vi "LED-Testing-JAP_v8.vi"() -> ()   [LabVIEW 2018]
uses:
  <vilib>/Utility/file.llb/Write Delimited Spreadsheet (string).vi
  LED_Test_JAP/SubVIs_LED-Testing-JAP_v2/Keithley 24XX/Keithley 24XX.lvlib
panel:
  in  "Compl. 3 (A)":dbl=0.09
  in  "Volt for Comp. 3 (V)":dbl=4.0 format="%#_13g"
  in  "Compl. 1 (A)":dbl=0.0009
  in  "Compl. 2 (A)":dbl=0.009
  out "Test Current (A)":string
  in  "Test":bool
  in  "stop":bool
  in  "Test Voltage (V)":dbl=0.1
  in  "Voltage range (V)":enum16{"0.2", "2", "20", "200"}(ring)=enum."20"
  out "Spectrum":cluster{"Y":dbl[], "Y":dbl[]}[](graph)
  out "L-V":cluster{"Y":dbl[], "Y":dbl[]}[](graph)
  out "Current efficiency - V":cluster{"Y":dbl[], "Y":dbl[]}[](graph)
  in  "Step 2 (V)":dbl=0.5 format="%#_13g"
  in  "End (V)":dbl=15.0 format="%#_13g"
  out "Voltage (V) 2":dbl
  out "Current (A) 2":string
  out "Exp. Meas. Time 2":string
  out "Meas. complete 2":string
  out "Data - x, y, Lv 2":dbl[](array[numeric])
  out "Spectrum (380-780nm) 2":dbl[](array[numeric])
  in  "Mode 2":enum16{"iV", "iVL"}(ring)=enum."iVL"
  in  "Interval 2 (ms)":dbl=500.0
  in  "Mode 1":enum16{"iV", "iVL"}(ring)
  in  "?":enum32{"Results", "Spectra"}(tab)
  out "Area (mm2), Voltage (V),  Current (A), Current density (mA/cm2), Current efficiency (Cd/A), Luminance (Cd/m2), CIEx, CIEy":ext[][](array[numeric])
  out "Spectral radiant intensity at different voltages (header)":ext[][](array[numeric])
  out "Spectrum (380-780nm)":dbl[](array[numeric])
  out "Data - x, y, Lv":dbl[](array[numeric])
  out "Meas. complete":string
  out "Exp. Meas. Time":string
  in  "error in (no error)":errorcluster
  in  "CS-2000 VISA name":refnum<visa-resource-name>="COM3"
  out "error out 2":errorcluster
  in  "Compliance (A)":dbl=0.0009
  in  "Start (V)":dbl
  in  "Mid (V)":dbl=2.5 format="%#_13g"
  in  "Step 1 (V)":dbl=0.1 format="%#_13g"
  out "Voltage (V)":dbl
  out "Current (A)":string
  in  "Stop":bool
  out "J-V":cluster{"Y":dbl[], "Y":dbl[]}[](graph)
  in  "Pixel area (mm2)":dbl=4.5
  in  "Interval 1 (ms)":dbl=500.0
  in  "Directory:":path=path "C:/Users/Talapin Lab/Desktop/LED_Test_JAP/Data/Himchan/20180725"
  in  "File name:":string
  in  "Insert time stamp:":bool=TRUE
  in  "Quit":bool
  in  "Start":bool
  in  "Keithley2400 VISA name":refnum<visa-resource-name>="GPIB0::24::INSTR"
  # "Area (mm2)"
  # "Voltage (V)"
  # "Current (A)"
  # "Current density (mA/cm2)"
  # "Current efficiency (Cd/A)"
  # "Luminance \n(Cd/m2)"
  # "CIEx"
  # "CIEy"
  # "Wavelength (nm)"
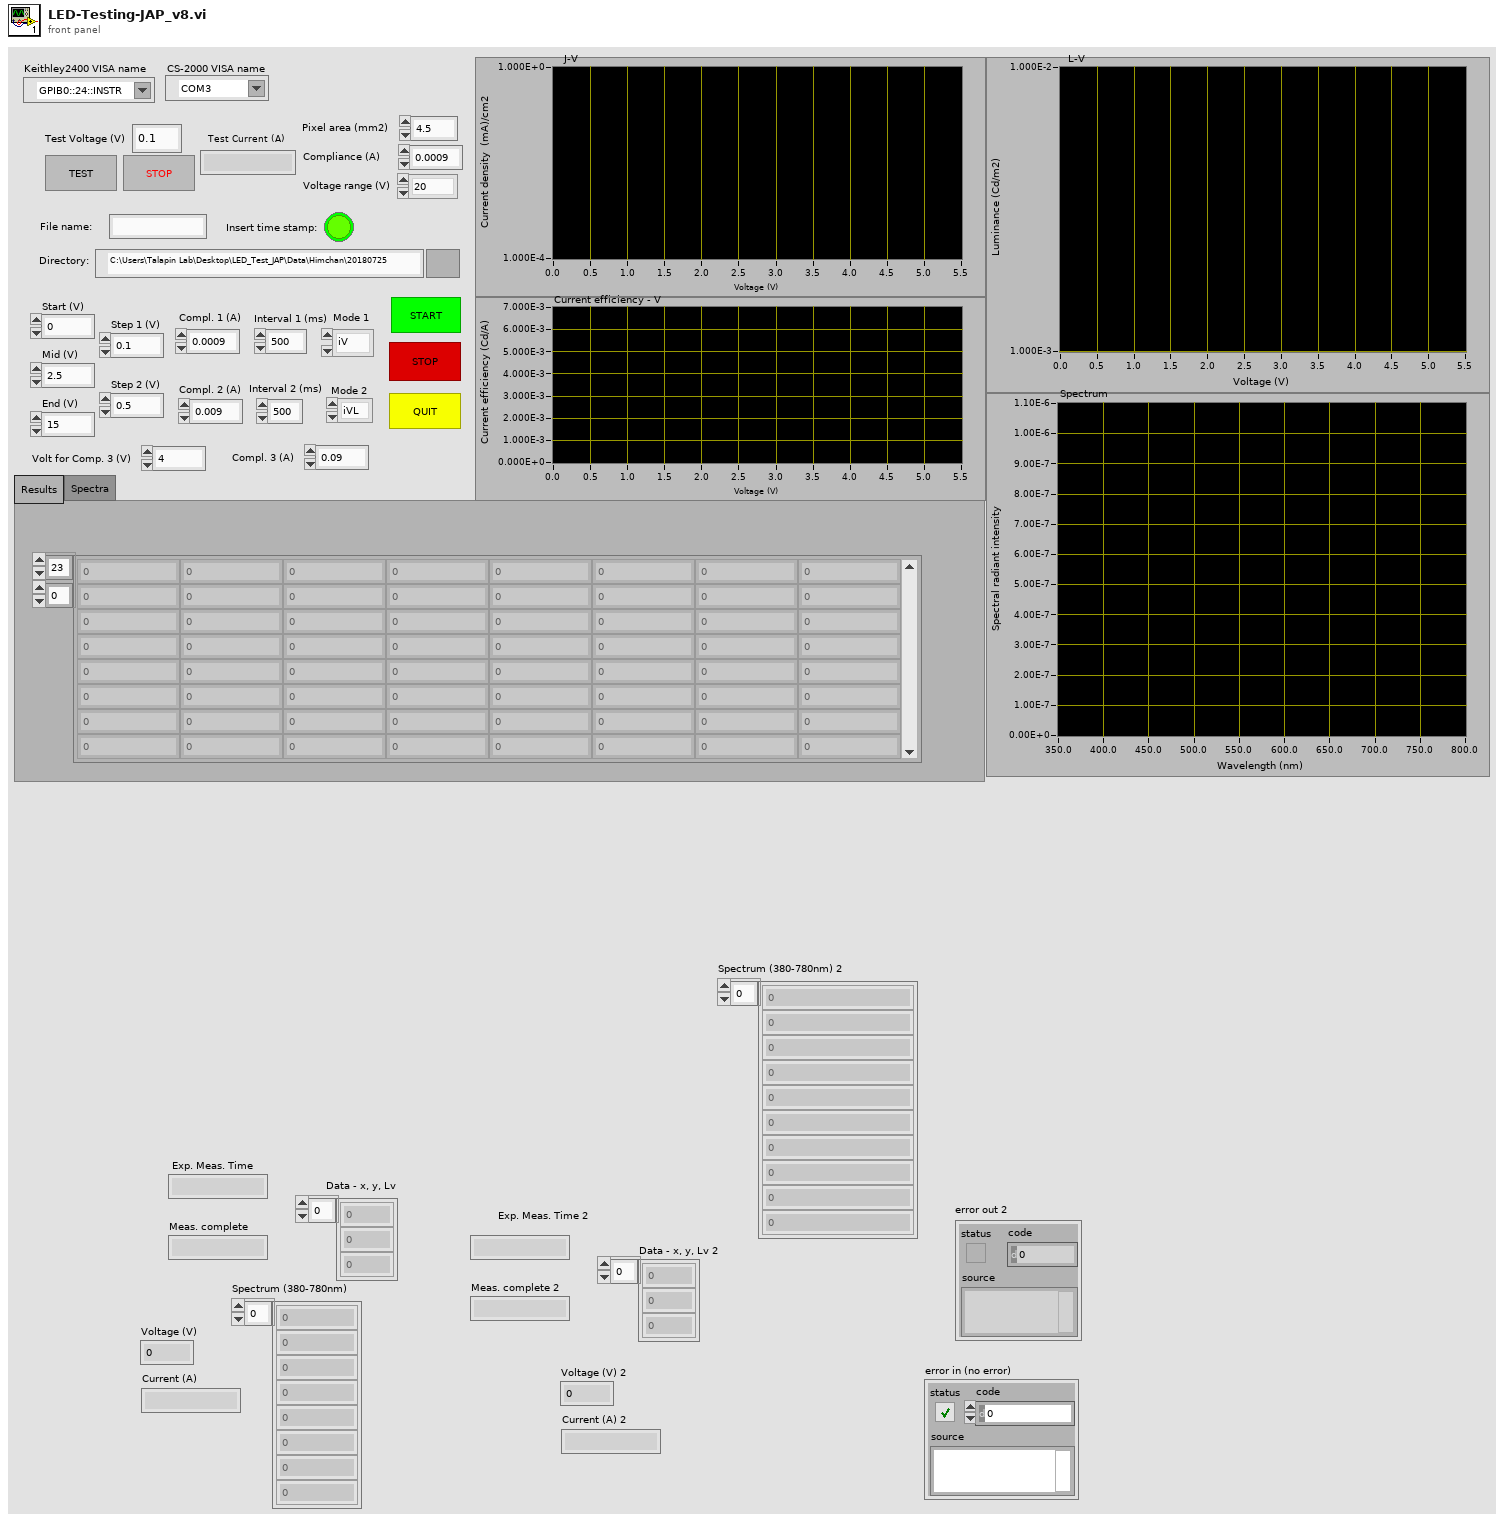
[diagram p1: front panel]
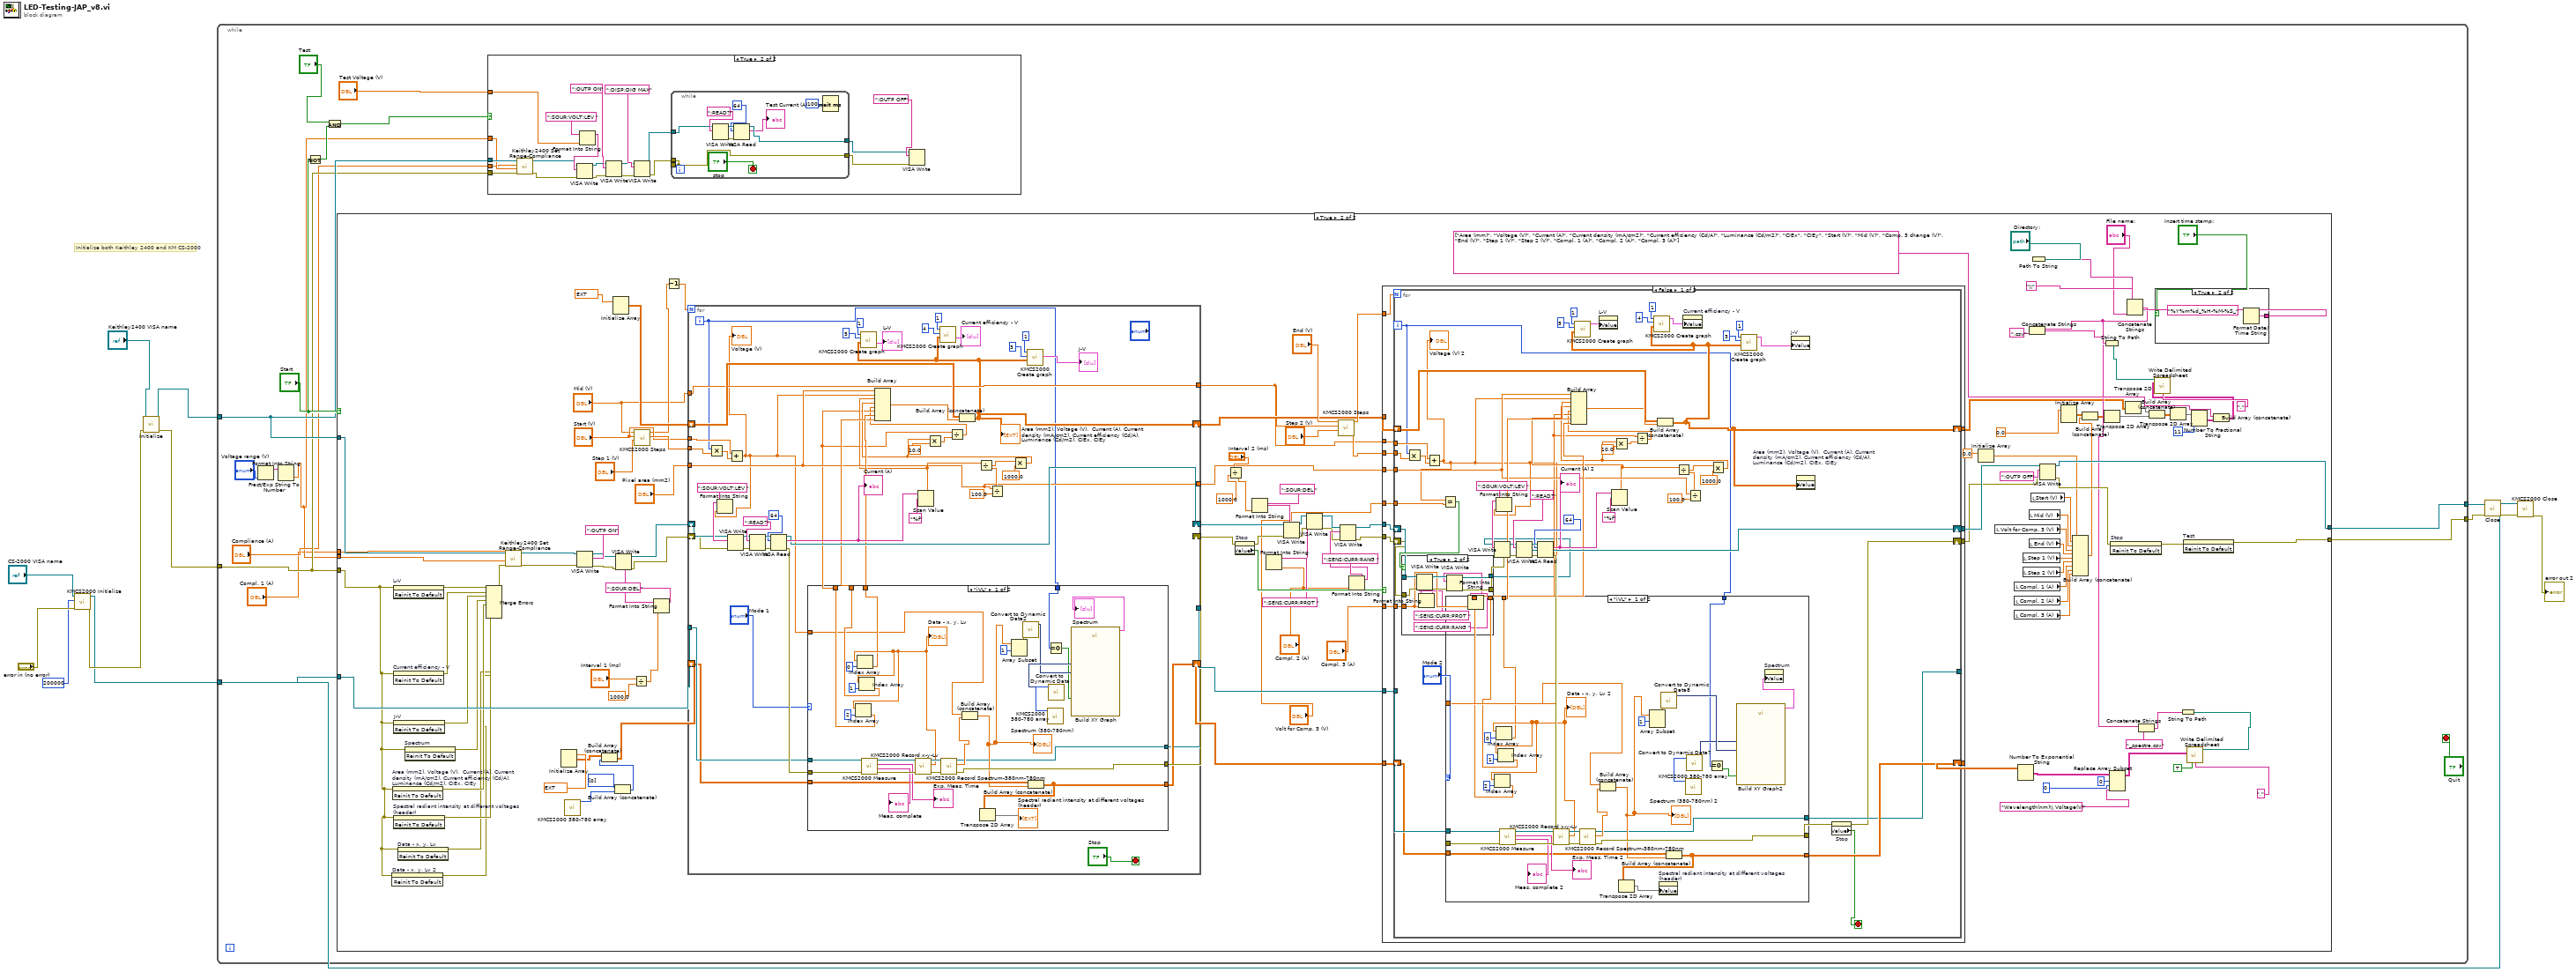
[diagram p0: block diagram]
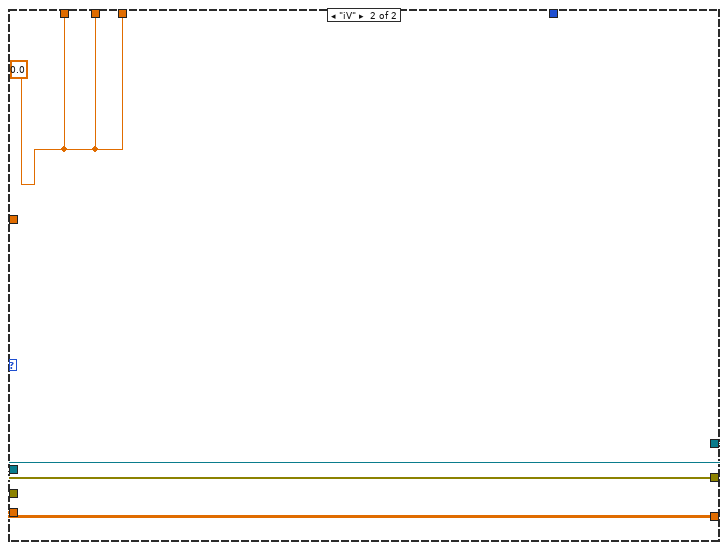
[diagram p5: hidden frame]
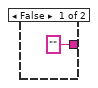
[diagram p7: hidden frame]
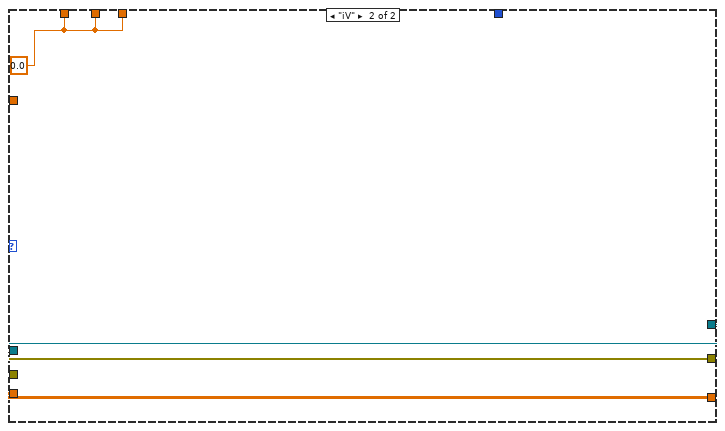
[diagram p8: hidden frame]
diagram:
  # "Initialize both Keithley 2400 and KM CS-2000"
  n1 = call "KMCS2000 Initialize.vi"("error in (no error)"="error in (no error)", "timeout (10sec)"=u32 200000, "VISA Refnum in"="CS-2000 VISA name") -> ("error out"=w5:errorcluster, "VISA Refnum out"=w2:refnum<visa-resource-name>)  [unwired: 7 in]
  n2 = call "Initialize.vi"("error in (no error)"=w5, "VISA resource name"="Keithley2400 VISA name") -> ("error out"=w10:errorcluster, "VISA resource name out"=w11:refnum<visa-resource-name>)  [unwired: 8 in]
  n3 = while {
    tunnel: w11 -> [w21]
    tunnel: w10 -> [w20]
    tunnel: [w28] -> w9
    tunnel: [w27] -> w8
    tunnel: w2 -> [w25]
    stop <- "Quit" stop-if-true
    n4 = Format Into String("Voltage range (V)") -> (resulting string=w17:string)  [unwired: 3 in, 1 out]
    n5 = Fract/Exp String To Number(string=w17) -> (number=w16:dbl)  [unwired: 3 in, 1 out]
    n6 = Not(x="Start") -> (.not. x?=w23:bool)
    n7 = And(x="Test", y=w23) -> (x .and. y?=w22:bool)
    n8 = case shown="True" "Start" {
      tunnel: w21 -> [w60 w185]
      tunnel: w20 -> [w59 w87]
      tunnel: [w60 w178] -> w28
      tunnel: [w59 w106] -> w27
      tunnel: w25 -> [_ w155]
      tunnel: w16 -> [_ w109]
      tunnel: "Compl. 1 (A)" -> [_ w108]
      frame False {
      }
      frame True {
        n9 = invoke on="Data - x, y, Lv 2" class="Arr (strict)" method="Reinit To Default"(error in=w87) -> (error out=w85:errorcluster)  [unwired: 2 in, 2 out]
        n10 = invoke on="Area (mm2), Voltage (V),  Current (A), Current density (mA/cm2), Current efficiency (Cd/A), Luminance (Cd/m2), CIEx, CIEy" class="Arr (strict)" method="Reinit To Default"(error in=w87) -> (error out=w100:errorcluster)  [unwired: 2 in, 2 out]
        n11 = invoke on="L-V" class="XYGraph (strict)" method="Reinit To Default"(error in=w87) -> (error out=w104:errorcluster)  [unwired: 2 in, 2 out]
        n12 = invoke on="Current efficiency - V" class="XYGraph (strict)" method="Reinit To Default"(error in=w87) -> (error out=w103:errorcluster)  [unwired: 2 in, 2 out]
        n13 = invoke on="J-V" class="XYGraph (strict)" method="Reinit To Default"(error in=w87) -> (error out=w102:errorcluster)  [unwired: 2 in, 2 out]
        n14 = invoke on="Spectral radiant intensity at different voltages (header)" class="Arr (strict)" method="Reinit To Default"(error in=w87) -> (error out=w99:errorcluster)  [unwired: 2 in, 2 out]
        n15 = invoke on="Data - x, y, Lv" class="Arr (strict)" method="Reinit To Default"(error in=w87) -> (error out=w86:errorcluster)  [unwired: 2 in, 2 out]
        n16 = invoke on="Spectrum" class="XYGraph (strict)" method="Reinit To Default"(error in=w87) -> (error out=w101:errorcluster)  [unwired: 2 in, 2 out]
        n17 = Merge Errors(w104, w103, w102, w101, w100, w99, w86, w85) -> (w105:errorcluster)
        n18 = call "Keithley2400 Set Range-Compliance.vi"("error in (no error)"=w105, "Voltage range (V)"=w109, "Compliance (A)"=w108, "VISA Refnum in"=w185) -> ("error out"=w166:errorcluster, "VISA Refnum out"=w171:refnum<visa-resource-name>)  [unwired: 6 in]
        n19 = Initialize Array(ext 0.0) -> (w153:ext[][])  [unwired: 2 out]
        n20 = call "KMCS2000 380-780 array.vi"() -> ("Array"=w144:i32[])  [unwired: 11 in]
        n21 = VISA Write(VISA resource name=w171, write buffer=":OUTP ON", error in (no error)=w166) -> (VISA resource name out=w170:refnum<visa-resource-name>, error out=w167:errorcluster)  [unwired: 1 out]
        n22 = Initialize Array(ext 0.0) -> (w180:ext[][])  [unwired: 2 out]
        n23 = Build Array (concatenate)(i32[] [0] ("array"), w144) -> (w145:i32[])
        n24 = Build Array (concatenate)(w153, w145) -> (w152:ext[][])
        n25 = Divide(x="Interval 1 (ms)", y=1000.0) -> (x/y=w174:dbl)
        n26 = call "KMCS2000 Steps.vi"("Step 1"="Step 1 (V)", "Start (V)"="Start (V)", "Mid (V)"="Mid (V)") -> ("Step sizeand direction"=w183:dbl, "Number of steps"=w117:dbl)  [unwired: 7 in]
        n27 = Format Into String(initial string=":SOUR:DEL " ("write buffer"), w174) -> (resulting string=w175:string)  [unwired: 2 in, 1 out]
        n28 = VISA Write(VISA resource name=w170, write buffer=w175, error in (no error)=w167) -> (VISA resource name out=w169:refnum<visa-resource-name>, error out=w168:errorcluster)  [unwired: 1 out]
        n29 = Decrement(x=w117) -> (x-1=w116:dbl)
        n30 = for {
          N: w116 -> [_]
          tunnel: w183 -> [w364]
          tunnel: "Start (V)" -> [w333]
          shift-right: [w315] -> w122
          shift-left: w180 -> [w362]
          shift-right: [w351] -> w130
          shift-left: w169 -> [w353]
          shift-right: [w340] -> w112
          shift-left: w168 -> [w352]
          tunnel: w155 -> [w341]
          shift-right: [w336] -> w124
          shift-left: w152 -> [w337]
          tunnel: "Pixel area (mm2)" -> [w330]
          tunnel: [w335] -> w123
          tunnel: [w330] -> w129
          tunnel: [w332] -> w118
          tunnel: "Mid (V)" -> [w332]
          i -> [w313]
          stop <- "Stop" stop-if-true
          n31 = Multiply(x=w313, y=w364) -> (x*y=w363:dbl)
          n32 = Add(x=w333, y=w363) -> (x+y=w329:dbl)
          "Voltage (V)" <- w329
          n33 = Format Into String(initial string=":SOUR:VOLT:LEV " ("write buffer"), w329) -> (resulting string=w359:string)  [unwired: 2 in, 1 out]
          n34 = VISA Write(VISA resource name=w353, write buffer=w359, error in (no error)=w352) -> (VISA resource name out=w354:refnum<visa-resource-name>, error out=w350:errorcluster)  [unwired: 1 out]
          n35 = VISA Write(VISA resource name=w354, write buffer=":READ?", error in (no error)=w350) -> (VISA resource name out=w357:refnum<visa-resource-name>, error out=w349:errorcluster)  [unwired: 1 out]
          n36 = VISA Read(VISA resource name=w357, byte count=u32 64, error in (no error)=w349) -> (VISA resource name out=w351:refnum<visa-resource-name>, read buffer=w356:string, error out=w342:errorcluster)  [unwired: 1 out]
          "Current (A)" <- w356
          n37 = case shown="\"iVL\"" "Mode 1" {
            tunnel: w342 -> [w386 w398]
            tunnel: w341 -> [w385 w396]
            tunnel: [w384 w398] -> w340
            tunnel: [w379 w399] -> w325
            tunnel: [w378 w399] -> w339
            tunnel: [w377 w399] -> w338
            tunnel: w337 -> [w376 w397]
            tunnel: [w375 w397] -> w336
            tunnel: w329 -> [w372 _]
            tunnel: [w368 w396] -> w335
            tunnel: w313 -> [w365 _]
            frame "iVL" {
              n38 = call "KMCS2000 Measure.vi"("error in (no error)"=w386, "VISA Refnum in"=w385) -> ("error out"=w394:errorcluster, "Meas. complete"=→"Meas. complete":string, "Exp. Meas. Time"=→"Exp. Meas. Time":string, "VISA Refnum out"=w395:refnum<visa-resource-name>)  [unwired: 6 in]
              n39 = call "KMCS2000 Record x-y-Lv.vi"("error in (no error)"=w394, "VISA Refnum in"=w395) -> ("error out"=w392:errorcluster, "Data - x, y, Lv"=w380:dbl[], "VISA Refnum out"=w393:refnum<visa-resource-name>)  [unwired: 7 in]
              "Data - x, y, Lv" <- w380
              n40 = Index Array(array=w380, index=2) -> (element=w379:dbl)
              n41 = Index Array(array=w380, index=0) -> (element=w378:dbl)
              n42 = Index Array(array=w380, index=1) -> (element=w377:dbl)
              n43 = call "KMCS2000 Record Spectrum-380nm-780nm.vi"("error in (no error)"=w392, "VISA Refnum in"=w393) -> ("error out"=w384:errorcluster, "Spectrum (380-780nm)"=w373:dbl[], "VISA Refnum out"=w368:refnum<visa-resource-name>)  [unwired: 7 in]
              n44 = Build Array (concatenate)(w372, w373) -> (w371:dbl[])
              "Spectrum (380-780nm)" <- w371
              n45 = Array Subset(array=w371, index=1) -> (w370:dbl[])  [unwired: 1 in]
              n46 = call "Convert to Dynamic Data2"("Array"=w370) -> ("Dynamic Data Type"=w387:dynamicdata)  [unwired: 3 in]
              n47 = Build Array (concatenate)(w376, w371) -> (w375:ext[][])
              n48 = Transpose 2D Array(2D array=w375) -> (transposed array=→"Spectral radiant intensity at different voltages (header)":ext[][])
              n49 = call "KMCS2000 380-780 array.vi"() -> ("Array"=w389:i32[])  [unwired: 11 in]
              n50 = Equal To 0?(x=w365) -> (x = 0?=w366:bool)
              n51 = call "Convert to Dynamic Data"("Array"=w389) -> ("Dynamic Data Type"=w388:dynamicdata)  [unwired: 3 in]
              n52 = call "Build XY Graph"("Reset"=w366, "Y Input"=w387, "X Input"=w388) -> ("XY Graph"=→"Spectrum":cluster{"X":dbl[], "Y":dbl[]}[])  [unwired: 7 in, 1 out]
            }
            frame "iV" {
              w399 = 0.0
            }
          }
          n53 = Scan Value(string=w356, format string="%f") -> (value=w328:dbl)  [unwired: 1 in, 1 out]
          n54 = Divide(x=w330, y=100.0) -> (x/y=w345:dbl)
          n55 = Divide(x=w328, y=w345) -> (x/y=w344:dbl)
          n56 = Multiply(x=w344, y=1000.0) -> (x*y=w327:dbl)
          n57 = Multiply(x=w327, y=10.0) -> (x*y=w324:dbl)
          n58 = Divide(x=w325, y=w324) -> (x/y=w323:dbl)
          n59 = Build Array(w330, w329, w328, w327, w323, w325, w339, w338) -> (w361:dbl[])
          n60 = Build Array (concatenate)(w362, w361) -> (w315:ext[][])
          "Area (mm2), Voltage (V),  Current (A), Current density (mA/cm2), Current efficiency (Cd/A), Luminance (Cd/m2), CIEx, CIEy" <- w315
          n61 = call "KMCS2000 Create graph.vi"("Array"=w315, "y index"=5 ("disabled index (col)"), "x index"=1 ("disabled index (col)")) -> ("XY Graph"=→"L-V":cluster{"X":dbl[], "Y":dbl[]}[])  [unwired: 8 in]
          n62 = call "KMCS2000 Create graph.vi"("Array"=w315, "y index"=4 ("disabled index (col)"), "x index"=1 ("disabled index (col)")) -> ("XY Graph"=→"Current efficiency - V":cluster{"X":dbl[], "Y":dbl[]}[])  [unwired: 8 in]
          n63 = call "KMCS2000 Create graph.vi"("Array"=w315, "y index"=3 ("disabled index (col)"), "x index"=1 ("disabled index (col)")) -> ("XY Graph"=→"J-V":cluster{"X":dbl[], "Y":dbl[]}[])  [unwired: 8 in]
        }
        n64 = Divide(x="Interval 2 (ms)", y=1000.0) -> (x/y=w134:dbl)
        n65 = property on="Stop" class="Bool (strict)"(error in=w112) -> (error out=w111:errorcluster, "Value"=w110:bool)  [unwired: 1 in, 1 out]
        n66 = Format Into String(initial string=":SOUR:DEL " ("write buffer"), w134) -> (resulting string=w131:string)  [unwired: 2 in, 1 out]
        n67 = Format Into String(initial string=":SENS:CURR:PROT " ("write buffer"), "Compl. 2 (A)") -> (resulting string=w96:string)  [unwired: 2 in, 1 out]
        n68 = VISA Write(VISA resource name=w130, write buffer=w131, error in (no error)=w111) -> (VISA resource name out=w91:refnum<visa-resource-name>, error out=w89:errorcluster)  [unwired: 1 out]
        n69 = VISA Write(VISA resource name=w91, write buffer=w96, error in (no error)=w89) -> (VISA resource name out=w93:refnum<visa-resource-name>, error out=w92:errorcluster)  [unwired: 1 out]
        n70 = call "KMCS2000 Steps.vi"("Step 1"="Step 2 (V)", "Start (V)"=w118, "Mid (V)"="End (V)") -> ("Step sizeand direction"=w126:dbl, "Number of steps"=w125:dbl)  [unwired: 7 in]
        n71 = Format Into String(initial string=":SENS:CURR:RANG " ("write buffer"), "Compl. 2 (A)") -> (resulting string=w95:string)  [unwired: 2 in, 1 out]
        n72 = VISA Write(VISA resource name=w93, write buffer=w95, error in (no error)=w92) -> (VISA resource name out=w90:refnum<visa-resource-name>, error out=w88:errorcluster)  [unwired: 1 out]
        n73 = case shown="False" w110 {
          tunnel: w129 -> [w200 _]
          tunnel: w126 -> [w199 _]
          tunnel: w125 -> [w198 _]
          tunnel: w124 -> [w197 w308]
          tunnel: w123 -> [w196 _]
          tunnel: w122 -> [w195 w309]
          tunnel: [w194 w309] -> w65
          tunnel: [w193 w306] -> w121
          tunnel: [w192 w307] -> w120
          tunnel: [w191 w308] -> w119
          tunnel: w118 -> [w190 _]
          tunnel: w90 -> [w189 w306]
          tunnel: w88 -> [w188 w307]
          tunnel: "Volt for Comp. 3 (V)" -> [w187 _]
          tunnel: "Compl. 3 (A)" -> [w186 _]
          frame False {
            n74 = for {
              N: w198 -> [_]
              tunnel: w199 -> [w257]
              tunnel: w190 -> [w256]
              shift-right: [w213] -> w194
              shift-left: w195 -> [w254]
              shift-right: [w244] -> w193
              shift-left: w189 -> [w205]
              shift-right: [w222] -> w192
              shift-left: w188 -> [w203]
              tunnel: w196 -> [w236]
              shift-right: [w232] -> w191
              shift-left: w197 -> [w233]
              tunnel: w200 -> [w229]
              tunnel: [w231] -> _
              tunnel: w187 -> [w207]
              tunnel: w186 -> [w201]
              i -> [w209]
              stop <- w220 stop-if-true
              n75 = Multiply(x=w209, y=w257) -> (x*y=w255:dbl)
              n76 = Add(x=w256, y=w255) -> (x+y=w208:dbl)
              "Voltage (V) 2" <- w208
              n77 = Equal?(x=w208, y=w207) -> (x = y?=w206:bool)
              n78 = case shown="True" w206 {
                tunnel: w205 -> [w259 w270]
                tunnel: [w259 w268] -> w204
                tunnel: w203 -> [w258 w267]
                tunnel: [w258 w265] -> w202
                tunnel: w201 -> [_ w264]
                frame False {
                }
                frame True {
                  n79 = Format Into String(initial string=":SENS:CURR:PROT " ("write buffer"), w264) -> (resulting string=w262:string)  [unwired: 2 in, 1 out]
                  n80 = VISA Write(VISA resource name=w270, write buffer=w262, error in (no error)=w267) -> (VISA resource name out=w269:refnum<visa-resource-name>, error out=w266:errorcluster)  [unwired: 1 out]
                  n81 = Format Into String(initial string=":SENS:CURR:RANG " ("write buffer"), w264) -> (resulting string=w260:string)  [unwired: 2 in, 1 out]
                  n82 = VISA Write(VISA resource name=w269, write buffer=w260, error in (no error)=w266) -> (VISA resource name out=w268:refnum<visa-resource-name>, error out=w265:errorcluster)  [unwired: 1 out]
                }
              }
              n83 = Format Into String(initial string=":SOUR:VOLT:LEV " ("write buffer"), w208) -> (resulting string=w251:string)  [unwired: 2 in, 1 out]
              n84 = VISA Write(VISA resource name=w204, write buffer=w251, error in (no error)=w202) -> (VISA resource name out=w245:refnum<visa-resource-name>, error out=w243:errorcluster)  [unwired: 1 out]
              n85 = VISA Write(VISA resource name=w245, write buffer=":READ?", error in (no error)=w243) -> (VISA resource name out=w249:refnum<visa-resource-name>, error out=w242:errorcluster)  [unwired: 1 out]
              n86 = VISA Read(VISA resource name=w249, byte count=u32 64, error in (no error)=w242) -> (VISA resource name out=w244:refnum<visa-resource-name>, read buffer=w247:string, error out=w237:errorcluster)  [unwired: 1 out]
              "Current (A) 2" <- w247
              n87 = case shown="\"iVL\"" "Mode 2" {
                tunnel: w237 -> [w294 w304]
                tunnel: w236 -> [w293 w302]
                tunnel: [w292 w304] -> w221
                tunnel: [w287 w305] -> w224
                tunnel: [w286 w305] -> w235
                tunnel: [w285 w305] -> w234
                tunnel: w233 -> [w284 w303]
                tunnel: [w283 w303] -> w232
                tunnel: w208 -> [w281 _]
                tunnel: [w277 w302] -> w231
                tunnel: w209 -> [w272 _]
                frame "iVL" {
                  n88 = call "KMCS2000 Measure.vi"("error in (no error)"=w294, "VISA Refnum in"=w293) -> ("error out"=w300:errorcluster, "Meas. complete"=→"Meas. complete 2":string, "Exp. Meas. Time"=→"Exp. Meas. Time 2":string, "VISA Refnum out"=w301:refnum<visa-resource-name>)  [unwired: 6 in]
                  n89 = call "KMCS2000 Record x-y-Lv.vi"("error in (no error)"=w300, "VISA Refnum in"=w301) -> ("error out"=w298:errorcluster, "Data - x, y, Lv"=w288:dbl[], "VISA Refnum out"=w299:refnum<visa-resource-name>)  [unwired: 7 in]
                  "Data - x, y, Lv 2" <- w288
                  n90 = Index Array(array=w288, index=2) -> (element=w287:dbl)
                  n91 = Index Array(array=w288, index=0) -> (element=w286:dbl)
                  n92 = Index Array(array=w288, index=1) -> (element=w285:dbl)
                  n93 = call "KMCS2000 Record Spectrum-380nm-780nm.vi"("error in (no error)"=w298, "VISA Refnum in"=w299) -> ("error out"=w292:errorcluster, "Spectrum (380-780nm)"=w282:dbl[], "VISA Refnum out"=w277:refnum<visa-resource-name>)  [unwired: 7 in]
                  n94 = Build Array (concatenate)(w281, w282) -> (w280:dbl[])
                  "Spectrum (380-780nm) 2" <- w280
                  n95 = Array Subset(array=w280, index=1) -> (w279:dbl[])  [unwired: 1 in]
                  n96 = call "Convert to Dynamic Data8"("Array"=w279) -> ("Dynamic Data Type"=w275:dynamicdata)  [unwired: 3 in]
                  n97 = Build Array (concatenate)(w284, w280) -> (w283:ext[][])
                  n98 = Transpose 2D Array(2D array=w283) -> (transposed array=w276:ext[][])
                  n99 = property on="Spectral radiant intensity at different voltages (header)" class="Arr (strict)"("Value"=w276) -> ()  [unwired: 2 in, 2 out]
                  n100 = call "KMCS2000 380-780 array.vi"() -> ("Array"=w295:i32[])  [unwired: 11 in]
                  n101 = call "Convert to Dynamic Data7"("Array"=w295) -> ("Dynamic Data Type"=w274:dynamicdata)  [unwired: 3 in]
                  n102 = Equal To 0?(x=w272) -> (x = 0?=w271:bool)
                  n103 = call "Build XY Graph2"("Reset"=w271, "Y Input"=w275, "X Input"=w274) -> ("XY Graph"=w273:cluster{"X":dbl[], "Y":dbl[]}[])  [unwired: 7 in, 1 out]
                  n104 = property on="Spectrum" class="XYGraph (strict)"("Value"=w273) -> ()  [unwired: 2 in, 2 out]
                }
                frame "iV" {
                  w305 = 0.0
                }
              }
              n105 = Scan Value(string=w247, format string="%f") -> (value=w228:dbl)  [unwired: 1 in, 1 out]
              n106 = Divide(x=w229, y=100.0) -> (x/y=w240:dbl)
              n107 = Divide(x=w228, y=w240) -> (x/y=w239:dbl)
              n108 = Multiply(x=w239, y=1000.0) -> (x*y=w227:dbl)
              n109 = Multiply(x=w227, y=10.0) -> (x*y=w225:dbl)
              n110 = Divide(x=w224, y=w225) -> (x/y=w223:dbl)
              n111 = Build Array(w229, w208, w228, w227, w223, w224, w235, w234) -> (w253:dbl[])
              n112 = Build Array (concatenate)(w254, w253) -> (w213:ext[][])
              n113 = call "KMCS2000 Create graph.vi"("Array"=w213, "y index"=5 ("disabled index (col)"), "x index"=1 ("disabled index (col)")) -> ("XY Graph"=w210:cluster{"X":dbl[], "Y":dbl[]}[])  [unwired: 8 in]
              n114 = property on="L-V" class="XYGraph (strict)"("Value"=w210) -> ()  [unwired: 2 in, 2 out]
              n115 = call "KMCS2000 Create graph.vi"("Array"=w213, "y index"=4 ("disabled index (col)"), "x index"=1 ("disabled index (col)")) -> ("XY Graph"=w211:cluster{"X":dbl[], "Y":dbl[]}[])  [unwired: 8 in]
              n116 = property on="Current efficiency - V" class="XYGraph (strict)"("Value"=w211) -> ()  [unwired: 2 in, 2 out]
              n117 = call "KMCS2000 Create graph.vi"("Array"=w213, "y index"=3 ("disabled index (col)"), "x index"=1 ("disabled index (col)")) -> ("XY Graph"=w212:cluster{"X":dbl[], "Y":dbl[]}[])  [unwired: 8 in]
              n118 = property on="J-V" class="XYGraph (strict)"("Value"=w212) -> ()  [unwired: 2 in, 2 out]
              n119 = property on="Area (mm2), Voltage (V),  Current (A), Current density (mA/cm2), Current efficiency (Cd/A), Luminance (Cd/m2), CIEx, CIEy" class="Arr (strict)"("Value"=w213) -> ()  [unwired: 2 in, 2 out]
              n120 = property on="Stop" class="Bool (strict)"(error in=w221) -> (error out=w222:errorcluster, "Value"=w220:bool)  [unwired: 1 in, 1 out]
            }
          }
          frame True {
          }
        }
        n121 = Initialize Array(0.0 ("element")) -> (w80:dbl[])  [unwired: 1 in]
        n122 = local read "Volt for Comp. 3 (V)"() -> (w75:dbl)
        n123 = local read "Compl. 1 (A)"() -> (w71:dbl)
        n124 = local read "Compl. 2 (A)"() -> (w70:dbl)
        n125 = local read "Compl. 3 (A)"() -> (w69:dbl)
        n126 = Number To Exponential String(number=w119) -> (E-format string=w137:string[][])  [unwired: 3 in]
        n127 = local read "Step 1 (V)"() -> (w73:dbl)
        n128 = local read "Step 2 (V)"() -> (w72:dbl)
        n129 = local read "Mid (V)"() -> (w76:dbl)
        n130 = local read "End (V)"() -> (w74:dbl)
        n131 = Path To String(path="Directory:") -> (string=w160:string)
        n132 = local read "Start (V)"() -> (w77:dbl)
        n133 = VISA Write(VISA resource name=w121, write buffer=":OUTP OFF", error in (no error)=w120) -> (VISA resource name out=w178:refnum<visa-resource-name>, error out=w115:errorcluster)  [unwired: 1 out]
        n134 = Initialize Array(0.0 ("element")) -> (w79:dbl[][])  [unwired: 2 in]
        n135 = Build Array (concatenate)(w80, w77, w76, w75, w74, w73, w72, w71, w70, w69) -> (w78:dbl[])
        n136 = Build Array (concatenate)(w79, w78) -> (w64:dbl[][])
        n137 = Transpose 2D Array(2D array=w64) -> (transposed array=w67:dbl[][])
        n138 = Replace Array Subset(array=w137, new element="Wavelength(nm)\\ Voltage(V)" ("new element/subarray"), index (row)=0, index (col)=0 ("disabled index (col)")) -> (w139:string[][])
        n139 = invoke on="Stop" class="Bool (strict)" method="Reinit To Default"(error in=w115) -> (error out=w107:errorcluster)  [unwired: 2 in, 2 out]
        n140 = Transpose 2D Array(2D array=w65) -> (transposed array=w68:ext[][])
        n141 = Build Array (concatenate)(w68, w67) -> (w66:ext[][])
        n142 = case shown="True" "Insert time stamp:" {
          tunnel: ["" ("date/time string") w311] -> w159
          frame False {
          }
          frame True {
            n143 = Format Date/Time String(time format string (%c)="%Y%m%d_%H-%M-%S_") -> (date/time string=w311:string)  [unwired: 2 in]
          }
        }
        n144 = Concatenate Strings(w160, "\\" ("string"), w159, "File name:") -> (w114:string)
        n145 = Concatenate Strings(w114, ".csv" ("string")) -> (w149:string)
        n146 = String To Path(string=w149) -> (path=w162:path)
        n147 = Concatenate Strings(w114, "_spectra.csv" ("string")) -> (w146:string)
        n148 = Transpose 2D Array(2D array=w66) -> (transposed array=w62:ext[][])
        n149 = String To Path(string=w146) -> (path=w147:path)
        n150 = invoke on="Test" class="Bool" method="Reinit To Default"(error in=w107) -> (error out=w106:errorcluster)  [unwired: 2 in, 2 out]
        n151 = call-poly <vilib>:"Write Delimited Spreadsheet.vi"("file path (dialog if empty)"=w147, "2D data"=w139, "transpose? (no:F)"=TRUE, "delimiter (\\t)"="," ("delimiter (\\t)")) -> ()  [unwired: 10 in, 2 out]
        n152 = Number To Fractional String(number=w62, precision (6)=i16 11) -> (F-format string=w63:string[][])  [unwired: 2 in]
        n153 = Build Array (concatenate)(string[] ["Area (mm)", "Voltage (V)", "Current (A)", "Current density (mA/cm2)", "Current efficiency (Cd/A)", "Luminance (Cd/m2)", "CIEx", "CIEy", "Start (V)", "Mid (V)", "Comp. 3 change (V)", "End (V)", "Step 1 (V)", "Step 2 (V)", "Compl. 1 (A)", "Compl. 2 (A)", "Compl. 3 (A)"], w63) -> (w163:string[][])
        n154 = call-poly <vilib>:"Write Delimited Spreadsheet.vi"("file path (dialog if empty)"=w162, "2D data"=w163, "delimiter (\\t)"="," ("delimiter (\\t)")) -> ()  [unwired: 11 in, 2 out]
      }
    }
    n155 = case shown="True" w22 {
      tunnel: w21 -> [_ w48]
      tunnel: w20 -> [_ w47]
      tunnel: w16 -> [_ w46]
      tunnel: "Compliance (A)" -> [_ w45]
      tunnel: "Test Voltage (V)" -> [_ w42]
      frame False {
      }
      frame True {
        n156 = call "Keithley2400 Set Range-Compliance.vi"("error in (no error)"=w47, "Voltage range (V)"=w46, "Compliance (A)"=w45, "VISA Refnum in"=w48) -> ("error out"=w40:errorcluster, "VISA Refnum out"=w41:refnum<visa-resource-name>)  [unwired: 6 in]
        n157 = Format Into String(initial string=":SOUR:VOLT:LEV " ("write buffer"), w42) -> (resulting string=w44:string)  [unwired: 2 in, 1 out]
        n158 = VISA Write(VISA resource name=w41, write buffer=w44, error in (no error)=w40) -> (VISA resource name out=w38:refnum<visa-resource-name>, error out=w37:errorcluster)  [unwired: 1 out]
        n159 = VISA Write(VISA resource name=w38, write buffer=":OUTP ON", error in (no error)=w37) -> (VISA resource name out=w30:refnum<visa-resource-name>, error out=w29:errorcluster)  [unwired: 1 out]
        n160 = VISA Write(VISA resource name=w30, write buffer=":DISP:DIG MAX", error in (no error)=w29) -> (VISA resource name out=w32:refnum<visa-resource-name>, error out=w31:errorcluster)  [unwired: 1 out]
        n161 = while {
          tunnel: w32 -> [w52]
          tunnel: [w49] -> _
          tunnel: [w51] -> w35
          tunnel: [w49] -> w34
          tunnel: w31 -> [w49]
          stop <- "stop" stop-if-true
          n162 = VISA Write(VISA resource name=w52, write buffer=":READ?") -> (VISA resource name out=w56:refnum<visa-resource-name>, error out=w55:errorcluster)  [unwired: 1 in, 1 out]
          n163 = VISA Read(VISA resource name=w56, byte count=u32 64, error in (no error)=w55) -> (VISA resource name out=w51:refnum<visa-resource-name>, read buffer=→"Test Current (A)":string)  [unwired: 2 out]
          n164 = Wait (ms)(milliseconds to wait=u32 100) -> ()  [unwired: 1 out]
        }
        n165 = VISA Write(VISA resource name=w35, write buffer=":OUTP OFF", error in (no error)=w34) -> ()  [unwired: 3 out]
      }
    }
  }
  n166 = call "Close.vi"("error in (no error)"=w8, "VISA resource name"=w9) -> ("error out"=w4:errorcluster)  [unwired: 9 in]
  n167 = call "KMCS2000 Close.vi"("error in (no error)"=w4, "VISA Refnum in"=w2) -> ("error out"=→"error out 2":errorcluster)  [unwired: 9 in]
